vi "Efficiency Plot Main.vi"(0 "SMU 1 (Source)":refnum<k15>="4139_1", 1 "Voltage Steps":dbl[](array[numeric])=[8.5, 12.0, 24.0, 36.0, 48.0, 60.0], 5 "SMU 2 (Sink)":refnum<k15>="4139_2", 7 "Current Sweep Start":dbl format="%0.2f", 9 "Current Sweep End":dbl=-3.0 format="%0.2f", 11 "Error In":errorcluster, 12 "# Points":i32=50) -> (6 "Efficiency Plot":cluster{"current measurements":dbl[], dbl[]}[](graph)=[{"current measurements"=[0.0, 0.061224489795918366, 0.12244897959183673, 0.1836734693877551, 0.24489795918367346, 0.30612244897959184, 0.3673469387755102, 0.42857142857142855, 0.4897959183673469, 0.5510204081632653, 0.6122448979591837, 0.673469387755102, 0.7346938775510204, 0.7959183673469388, 0.8571428571428571, 0.9183673469387755, 0.9795918367346939, 1.0408163265306123, 1.1020408163265305, 1.163265306122449, 1.2244897959183674, 1.2857142857142858, 1.346938775510204, 1.4081632653061225, 1.469387755102041, 1.530612244897959, 1.5918367346938775, 1.653061224489796, 1.7142857142857142, 1.7755102040816326, 1.836734693877551, 1.8979591836734695, 1.9591836734693877, 2.020408163265306, 2.0816326530612246, 2.142857142857143, 2.204081632653061, 2.2653061224489797, 2.326530612244898, 2.3877551020408165, 2.4489795918367347, 2.510204081632653, 2.5714285714285716, 2.63265306122449, 2.693877551020408, 2.7551020408163267, 2.816326530612245, 2.877551020408163, 2.938775510204082, 3.0], [nan, inf, inf, inf, inf, inf, inf, inf, inf, inf, inf, inf, inf, inf, inf, inf, inf, inf, inf, inf, inf, inf, inf, inf, inf, inf, inf, inf, inf, inf, inf, inf, inf, inf, inf, inf, inf, inf, inf, inf, inf, inf, inf, inf, inf, inf, inf, inf, inf, inf]}, {"current measurements"=[0.0, 0.061224489795918366, 0.12244897959183673, 0.1836734693877551, 0.24489795918367346, 0.30612244897959184, 0.3673469387755102, 0.42857142857142855, 0.4897959183673469, 0.5510204081632653, 0.6122448979591837, 0.673469387755102, 0.7346938775510204, 0.7959183673469388, 0.8571428571428571, 0.9183673469387755, 0.9795918367346939, 1.0408163265306123, 1.1020408163265305, 1.163265306122449, 1.2244897959183674, 1.2857142857142858, 1.346938775510204, 1.4081632653061225, 1.469387755102041, 1.530612244897959, 1.5918367346938775, 1.653061224489796, 1.7142857142857142, 1.7755102040816326, 1.836734693877551, 1.8979591836734695, 1.9591836734693877, 2.020408163265306, 2.0816326530612246, 2.142857142857143, 2.204081632653061, 2.2653061224489797, 2.326530612244898, 2.3877551020408165, 2.4489795918367347, 2.510204081632653, 2.5714285714285716, 2.63265306122449, 2.693877551020408, 2.7551020408163267, 2.816326530612245, 2.877551020408163, 2.938775510204082, 3.0], [nan, inf, inf, inf, inf, inf, inf, inf, inf, inf, inf, inf, inf, inf, inf, inf, inf, inf, inf, inf, inf, inf, inf, inf, inf, inf, inf, inf, inf, inf, inf, inf, inf, inf, inf, inf, inf, inf, inf, inf, inf, inf, inf, inf, inf, inf, inf, inf, inf, inf]}, {"current measurements"=[0.0, 0.061224489795918366, 0.12244897959183673, 0.1836734693877551, 0.24489795918367346, 0.30612244897959184, 0.3673469387755102, 0.42857142857142855, 0.4897959183673469, 0.5510204081632653, 0.6122448979591837, 0.673469387755102, 0.7346938775510204, 0.7959183673469388, 0.8571428571428571, 0.9183673469387755, 0.9795918367346939, 1.0408163265306123, 1.1020408163265305, 1.163265306122449, 1.2244897959183674, 1.2857142857142858, 1.346938775510204, 1.4081632653061225, 1.469387755102041, 1.530612244897959, 1.5918367346938775, 1.653061224489796, 1.7142857142857142, 1.7755102040816326, 1.836734693877551, 1.8979591836734695, 1.9591836734693877, 2.020408163265306, 2.0816326530612246, 2.142857142857143, 2.204081632653061, 2.2653061224489797, 2.326530612244898, 2.3877551020408165, 2.4489795918367347, 2.510204081632653, 2.5714285714285716, 2.63265306122449, 2.693877551020408, 2.7551020408163267, 2.816326530612245, 2.877551020408163, 2.938775510204082, 3.0], [nan, inf, inf, inf, inf, inf, inf, inf, inf, inf, inf, inf, inf, inf, inf, inf, inf, inf, inf, inf, inf, inf, inf, inf, inf, inf, inf, inf, inf, inf, inf, inf, inf, inf, inf, inf, inf, inf, inf, inf, inf, inf, inf, inf, inf, inf, inf, inf, inf, inf]}, {"current measurements"=[0.0, 0.061224489795918366, 0.12244897959183673, 0.1836734693877551, 0.24489795918367346, 0.30612244897959184, 0.3673469387755102, 0.42857142857142855, 0.4897959183673469, 0.5510204081632653, 0.6122448979591837, 0.673469387755102, 0.7346938775510204, 0.7959183673469388, 0.8571428571428571, 0.9183673469387755, 0.9795918367346939, 1.0408163265306123, 1.1020408163265305, 1.163265306122449, 1.2244897959183674, 1.2857142857142858, 1.346938775510204, 1.4081632653061225, 1.469387755102041, 1.530612244897959, 1.5918367346938775, 1.653061224489796, 1.7142857142857142, 1.7755102040816326, 1.836734693877551, 1.8979591836734695, 1.9591836734693877, 2.020408163265306, 2.0816326530612246, 2.142857142857143, 2.204081632653061, 2.2653061224489797, 2.326530612244898, 2.3877551020408165, 2.4489795918367347, 2.510204081632653, 2.5714285714285716, 2.63265306122449, 2.693877551020408, 2.7551020408163267, 2.816326530612245, 2.877551020408163, 2.938775510204082, 3.0], [nan, inf, inf, inf, inf, inf, inf, inf, inf, inf, inf, inf, inf, inf, inf, inf, inf, inf, inf, inf, inf, inf, inf, inf, inf, inf, inf, inf, inf, inf, inf, inf, inf, inf, inf, inf, inf, inf, inf, inf, inf, inf, inf, inf, inf, inf, inf, inf, inf, inf]}, {"current measurements"=[0.0, 0.061224489795918366, 0.12244897959183673, 0.1836734693877551, 0.24489795918367346, 0.30612244897959184, 0.3673469387755102, 0.42857142857142855, 0.4897959183673469, 0.5510204081632653, 0.6122448979591837, 0.673469387755102, 0.7346938775510204, 0.7959183673469388, 0.8571428571428571, 0.9183673469387755, 0.9795918367346939, 1.0408163265306123, 1.1020408163265305, 1.163265306122449, 1.2244897959183674, 1.2857142857142858, 1.346938775510204, 1.4081632653061225, 1.469387755102041, 1.530612244897959, 1.5918367346938775, 1.653061224489796, 1.7142857142857142, 1.7755102040816326, 1.836734693877551, 1.8979591836734695, 1.9591836734693877, 2.020408163265306, 2.0816326530612246, 2.142857142857143, 2.204081632653061, 2.2653061224489797, 2.326530612244898, 2.3877551020408165, 2.4489795918367347, 2.510204081632653, 2.5714285714285716, 2.63265306122449, 2.693877551020408, 2.7551020408163267, 2.816326530612245, 2.877551020408163, 2.938775510204082, 3.0], [nan, inf, inf, inf, inf, inf, inf, inf, inf, inf, inf, inf, inf, inf, inf, inf, inf, inf, inf, inf, inf, inf, inf, inf, inf, inf, inf, inf, inf, inf, inf, inf, inf, inf, inf, inf, inf, inf, inf, inf, inf, inf, inf, inf, inf, inf, inf, inf, inf, inf]}, {"current measurements"=[0.0, 0.061224489795918366, 0.12244897959183673, 0.1836734693877551, 0.24489795918367346, 0.30612244897959184, 0.3673469387755102, 0.42857142857142855, 0.4897959183673469, 0.5510204081632653, 0.6122448979591837, 0.673469387755102, 0.7346938775510204, 0.7959183673469388, 0.8571428571428571, 0.9183673469387755, 0.9795918367346939, 1.0408163265306123, 1.1020408163265305, 1.163265306122449, 1.2244897959183674, 1.2857142857142858, 1.346938775510204, 1.4081632653061225, 1.469387755102041, 1.530612244897959, 1.5918367346938775, 1.653061224489796, 1.7142857142857142, 1.7755102040816326, 1.836734693877551, 1.8979591836734695, 1.9591836734693877, 2.020408163265306, 2.0816326530612246, 2.142857142857143, 2.204081632653061, 2.2653061224489797, 2.326530612244898, 2.3877551020408165, 2.4489795918367347, 2.510204081632653, 2.5714285714285716, 2.63265306122449, 2.693877551020408, 2.7551020408163267, 2.816326530612245, 2.877551020408163, 2.938775510204082, 3.0], [nan, inf, inf, inf, inf, inf, inf, inf, inf, inf, inf, inf, inf, inf, inf, inf, inf, inf, inf, inf, inf, inf, inf, inf, inf, inf, inf, inf, inf, inf, inf, inf, inf, inf, inf, inf, inf, inf, inf, inf, inf, inf, inf, inf, inf, inf, inf, inf, inf, inf]}], 15 "Error Out":errorcluster)   [LabVIEW 2014]
doc: "Demonstrates how to use triggers and events to synchronize multiple channels in Sequence source mode. Use this example to sequence multiple channels in lock-step."
uses:
  <instrlib>/niDCPower/nidcpower.llb/niDCPower Output Function.ctl
  <instrlib>/niDCPower/nidcpower.llb/niDCPower Source Mode.ctl
  <instrlib>/niDCPower/nidcpower.llb/niDCPower Sense.ctl
  <instrlib>/niDCPower/nidcpower.llb/niDCPower Sequence Attribute Type.ctl
  <instrlib>/niDCPower/nidcpower.llb/niDCPower Disable Source Trigger.vi
  <instrlib>/niDCPower/nidcpower.llb/niDCPower Configure Digital Edge Source Trigger.vi
  <instrlib>/niDCPower/nidcpower.llb/niDCPower Configure Digital Edge Measure Trigger.vi
panel:
  out "Input Voltage":cluster{"current measurements":dbl[], dbl[]}[](graph)=[{"current measurements"=[0.0037055805732003674, 0.06122110398172464, 0.12244845565372843, 0.18367430714253996, 0.24489790835656308, 0.30612338479957657, 0.3673477361051958, 0.42857227493371414, 0.48979531357904005, 0.5510198524075584, 0.6122447662818747, 0.673469305110393, 0.7346947815534065, 0.7959172576300354, 0.857143859210443, 0.9183685855618604, 0.9795921867758836, 1.0408167256044016, 1.102040139295526, 1.1632659907843375, 1.2244892169525623, 1.285714130826879, 1.3469392322240943, 1.4081635835297135, 1.4693883098811307, 1.5306113485264567, 1.5918375750610665, 1.6530617388437865, 1.7142855275807087, 1.7755106289779243, 1.8367346052377453, 1.8979597066349607, 1.9591831203260848, 2.0204080342004014, 2.0816321979831214, 2.1428574869032357, 2.204081838208855, 2.265305814468676, 2.3265305408200936, 2.387755642217309, 2.448979430954231, 2.5102045323514464, 2.571428696134167, 2.632652672393988, 2.693877586268304, 2.75510268766552, 2.8163259138337446, 2.877551390276758, 2.9387749914907815, 3.0000000928879964], [19.29819394334798, 86.6520550767066, 89.1654412635221, 91.38533524327332, 91.50919660281357, 92.04751308332489, 92.33568575131514, 92.46037426727128, 92.47606005503741, 92.42123593490287, 92.31633388123458, 92.17328677567859, 92.0042087848853, 91.81449657528333, 91.60799389168226, 91.38693943759473, 91.15523608809022, 90.91418462998905, 90.66679244318738, 90.41242663064665, 90.15379458586094, 89.89035373889821, 89.62363196341397, 89.35443181493694, 89.0829213803808, 88.80907867441277, 88.53272214141926, 88.25601431857473, 87.97816171947375, 87.69877401847535, 87.41899688296768, 87.13793625680408, 86.8562096461585, 86.57443041220006, 86.29187961010945, 86.0089768110029, 85.72632265506134, 85.4430679771896, 85.15955759219828, 84.87583568868575, 84.59217845404815, 84.30856400484413, 84.02480342907647, 83.74090983368129, 83.4569315652573, 83.17294308961198, 82.88907469498393, 82.6048754694049, 82.32014719341976, 82.03612720394379]}, {"current measurements"=[0.00021184144129742449, 0.06124941993947879, 0.12244864317662747, 0.18367468218833802, 0.24489772083366404, 0.30612282223087944, 0.36734661096780163, 0.4285726499795121, 0.4897964387164343, 0.5510209775449526, 0.6122447662818747, 0.6734694926332921, 0.7346942189847093, 0.7959183827674297, 0.8571419839814528, 0.9183672729015672, 0.9795906865926912, 1.0408157879899067, 1.102041076910021, 1.1632650531698423, 1.2244901545670577, 1.2857139433039797, 1.3469392322240943, 1.4081626459152183, 1.4693869972208375, 1.530611911095154, 1.5918370124923693, 1.6530621138895845, 1.7142855275807087, 1.775511004023722, 1.8367336676232504, 1.8979608317723549, 1.959183870417681, 2.02040634649431, 2.0816320104602224, 2.1428571118574378, 2.204080525548562, 2.265306189514474, 2.3265311033887905, 2.3877545170799146, 2.4489798060000294, 2.5102034072140524, 2.5714290711799648, 2.632653610008483, 2.693877586268304, 2.755102125096822, 2.8163259138337446, 2.877551765322556, 2.9387759291052764, 3.0000000928879964], [56.6452542558813, 80.64227031187568, 87.0782866841797, 86.4785053269065, 89.32488877347564, 88.67595189905475, 89.15300101728961, 89.59253187147004, 89.86482984693276, 90.01464408273661, 90.0842481389631, 90.0895693933995, 90.04935336193377, 89.97252157312707, 89.86619630761724, 89.73862887195637, 89.59305334468831, 89.43205240492902, 89.25985297739904, 89.07821163422473, 88.88761304096813, 88.68990824241101, 88.48605698427171, 88.2764978181229, 88.06295738097351, 87.84560283879459, 87.62562758853488, 87.40179887429976, 87.17616618084455, 86.94823753292036, 86.71826008167221, 86.4862789162294, 86.25326003643778, 86.01881763901763, 85.78341370157021, 85.54697019723872, 85.30945238666278, 85.07146384055599, 84.83237181630791, 84.59295584630685, 84.35280491363186, 84.11253310369847, 83.8713144132906, 83.63013754328348, 83.38832591662973, 83.14593896372894, 82.90348640956906, 82.66064568747939, 82.41734835561658, 82.17465456869868]}, {"current measurements"=[0.00023190639149405184, 0.06122616709999856, 0.12244845565372843, 0.18367299448224672, 0.24489790835656308, 0.30611963434159584, 0.3673464234449026, 0.4285713373192189, 0.4897964387164343, 0.5510202274533564, 0.6122443912360767, 0.6734694926332921, 0.7346936564160123, 0.7959187578132277, 0.8571427340730488, 0.9183668978557691, 0.9795916242071864, 1.0408159755128055, 1.102040889387122, 1.16326355298665, 1.2244895919983605, 1.285714130826879, 1.346939044701195, 1.4081630209610165, 1.4693877473124337, 1.5306117235722547, 1.5918360748778742, 1.6530615513208875, 1.7142855275807087, 1.775509691363429, 1.8367346052377453, 1.8979595191120617, 1.959183870417681, 2.020407096585906, 2.081631260368626, 2.1428571118574378, 2.204081463163057, 2.265305251899979, 2.3265301657742956, 2.387754892125713, 2.4489798060000294, 2.5102037822598504, 2.5714285086112674, 2.632653797531382, 2.693877961314102, 2.755102125096822, 2.8163264764024416, 2.8775504526622626, 2.93877517901368, 3.000000467933795], [24.507067975438325, 68.68728407459058, 75.82006753966498, 78.25552005826663, 80.46810288856278, 81.5286702792574, 83.9145213137586, 82.96197637388521, 83.64042372245805, 84.24184670017351, 84.68700598501955, 85.0119534280727, 85.2481904232033, 85.41356902440856, 85.52424026092518, 85.58780240316204, 85.61774812151559, 85.61373769771822, 85.58677874443494, 85.53768144152752, 85.47041365831792, 85.3885602534251, 85.29208143582215, 85.18407226185528, 85.06622105245873, 84.93930083598772, 84.80408544461643, 84.66242404506731, 84.51473417683798, 84.36085389725363, 84.2039049718862, 84.0407564161272, 83.87464336928115, 83.70526524132413, 83.53190139693746, 83.35600218690755, 83.17816187187974, 82.9976732670588, 82.81541633533251, 82.6305653803378, 82.44424776515379, 82.25691743396621, 82.06755259908867, 81.87689870447574, 81.68442031353618, 81.49075118570893, 81.29623828053742, 81.10028186493017, 80.90335145217146, 80.7055496663307]}, {"current measurements"=[0.00023828217006122054, 0.06122185407332076, 0.1224488306995265, 0.18367299448224672, 0.24489734578786596, 0.3061211345247881, 0.3673479236280948, 0.428571712365017, 0.4897960636706362, 0.5510207900220535, 0.6122449538047738, 0.673469680156191, 0.7346945940305074, 0.7959191328590258, 0.8571423590272509, 0.9183676479473653, 0.9795916242071864, 1.0408148503754115, 1.102040139295526, 1.1632652406927413, 1.2244903420899567, 1.285714318349778, 1.346938294609599, 1.4081628334381173, 1.4693868096979386, 1.5306109734806586, 1.5918364499236723, 1.6530624889353827, 1.7142851525349105, 1.775510066409227, 1.8367347927606443, 1.8979604567265569, 1.959183682894782, 2.0204087842919973, 2.0816327605518183, 2.1428571118574378, 2.2040816506859557, 2.265305814468676, 2.3265301657742956, 2.3877539545112176, 2.448979430954231, 2.5102047198743453, 2.5714273834738735, 2.63265229734819, 2.693877961314102, 2.7551017500510246, 2.816326663925341, 2.877551765322556, 2.938776491673974, 3.000000280410896], [15.625320952350052, 68.45323352659621, 68.41479018064763, 69.36918413162428, 75.8408948245319, 75.08515720349499, 78.57364834176967, 79.09049129203136, 78.79924593960071, 79.68628362365168, 80.3835328954986, 80.92405302473288, 81.34616501232134, 81.67333964560312, 81.92586994884321, 82.11470651158638, 82.25453463207786, 82.35150990030361, 82.41275896985898, 82.44583047463823, 82.45295390124451, 82.43852926466492, 82.40514186318386, 82.35672641765188, 82.2929138664694, 82.21790050512587, 82.13002218463713, 82.03354607731744, 81.92911100377732, 81.81594657215598, 81.6972655918749, 81.57150116100678, 81.44053403895059, 81.30463459966806, 81.16453795321308, 81.02039448531497, 80.87156952359493, 80.71958175528403, 80.56473166988907, 80.40678674122074, 80.2462075295369, 80.08317063844467, 79.91912233101111, 79.75064757843249, 79.58076401285685, 79.41032236358052, 79.23731818637971, 79.06327995782223, 78.88659495956507, 78.70957354063141]}, {"current measurements"=[0.0002388447387583213, 0.061227104714493726, 0.12244620537894002, 0.1836713067761554, 0.24490147129164477, 0.30612732278045623, 0.36734979885708513, 0.4285707747505218, 0.4897960636706362, 0.5510209775449526, 0.6122449538047738, 0.673468742541696, 0.7346945940305074, 0.7959187578132277, 0.8571429215959478, 0.91836671033287, 0.9795916242071864, 1.0408163505586037, 1.10204126443292, 1.1632656157385395, 1.2244910921815528, 1.285714130826879, 1.346938857178296, 1.4081624583923191, 1.4693881223582317, 1.530613598801245, 1.591835887354975, 1.6530611762750895, 1.7142855275807087, 1.775510816500823, 1.8367342301919474, 1.8979587690204656, 1.959183682894782, 2.0204085967690983, 2.0816323855060204, 2.1428574869032357, 2.20408090059436, 2.265306001991575, 2.3265297907284976, 2.3877547046028136, 2.448978868385534, 2.510203032168254, 2.571428883657066, 2.632652672393988, 2.6938772112225062, 2.7551023126197216, 2.816327414016937, 2.8775510152309596, 2.9387755540594784, 3.000000842979593], [10.685809147475581, 60.58664973802159, 69.32426572969297, 70.02017096472375, 70.60628775716478, 69.48609512689428, 73.16747403099501, 75.51894590720678, 74.45380140438738, 75.42803512625773, 76.3187834034888, 77.02711378666972, 77.591621229274, 78.04913495784959, 78.41201146737268, 78.7051508644127, 78.93314890895036, 79.11244376640121, 79.24599906988342, 79.3472307513215, 79.41532553446862, 79.45725266090052, 79.47501728817076, 79.47396673288904, 79.45412055016777, 79.41874717833805, 79.36947408129463, 79.30858436763418, 79.23748643871782, 79.15581950747247, 79.06485359860626, 78.96714312929933, 78.86342088702459, 78.75295744414646, 78.63548168504948, 78.51333325794127, 78.38617989431057, 78.25366220787029, 78.11974624015173, 77.98035710245406, 77.83837311795462, 77.69253126803493, 77.54419990931002, 77.39221211507345, 77.2389193042367, 77.08179535393343, 76.92307638925759, 76.76351534955948, 76.60023763509811, 76.43545824058003]}, {"current measurements"=[0.00023996987615252285, 0.061227104714493726, 0.12243795437138254, 0.18367468218833802, 0.24489997110845244, 0.30611813415840355, 0.3673460483991045, 0.42857096227342084, 0.4897926882584537, 0.5510215401136497, 0.6122455163734709, 0.6734700552019891, 0.7346947815534065, 0.7959180077216316, 0.8571429215959478, 0.9183674604244662, 0.9795919992529845, 1.0408165380815027, 1.102041076910021, 1.1632650531698423, 1.2244890294296633, 1.285713755781081, 1.3469375445180027, 1.4081637710526127, 1.4693866221750393, 1.53061266118675, 1.5918370124923693, 1.6530600511376952, 1.7142864651952041, 1.775510066409227, 1.8367347927606443, 1.8979595191120617, 1.959183870417681, 2.020407471631704, 2.0816335106434147, 2.1428572993803368, 2.204082025731754, 2.2653063770373736, 2.3265305408200936, 2.3877543295570156, 2.448979243431332, 2.5102049073972448, 2.5714285086112674, 2.632653234962685, 2.693877961314102, 2.7551008124365293, 2.816326663925341, 2.877551952845455, 2.938774428922084, 2.999999717842199], [8.037505223161133, 59.04402746018973, 65.93397111865757, 69.10832461216576, 69.88132934827026, 70.40864376659275, 71.07244623688928, 71.61813446388392, 70.88559085363639, 71.27919739280526, 72.31262277678016, 73.15099339025103, 73.83517876691829, 74.38997807165609, 74.8469795829111, 75.21574450005743, 75.51758140567794, 75.75633244380813, 75.94946682291643, 76.10238026373673, 76.21748823541188, 76.30401119763542, 76.36128741226422, 76.39717578408371, 76.4112319455966, 76.40815492818933, 76.38863918175531, 76.35552208706163, 76.31078311855917, 76.25546527873904, 76.18851950750565, 76.11259322339771, 76.02782989417233, 75.93726786864158, 75.84032284746705, 75.7354997513752, 75.62599197868968, 75.51069814477592, 75.39257747375275, 75.2695297016027, 75.14021925250529, 75.00917395178712, 74.87370939203441, 74.7357885393685, 74.59436663020796, 74.45166513872823, 74.30470438952655, 74.15585812945028, 74.00505290512945, 73.85269262177381]}]
  # "Sink"
  # "SOURCING OPERATION (SMU 1)\n1. Source Voltage Level and Fire Source Trigger Event \n2. Wait \"Delay\" Seconds\n3. Fire Source Complete Event\n3. Measure Current Immediately\n\nIV1, IV2, IV3...IV300 at V IN"
  # "SINKING OPERATION (SMU 2)\n1. Source Current Level (SMU1 Trigger)\n2. Wait \"Delay\" Seconds\n3. Measure Voltage (Using SMU1 Source Complete Event Trigger)\n\n\nIV1, IV2, IV3...IV300 at V OUT"
  # "Source"
  # "Iout = 0 to 3 A"
  # "Vin = 8 to 60 V"
  # "Vout = 5 V"
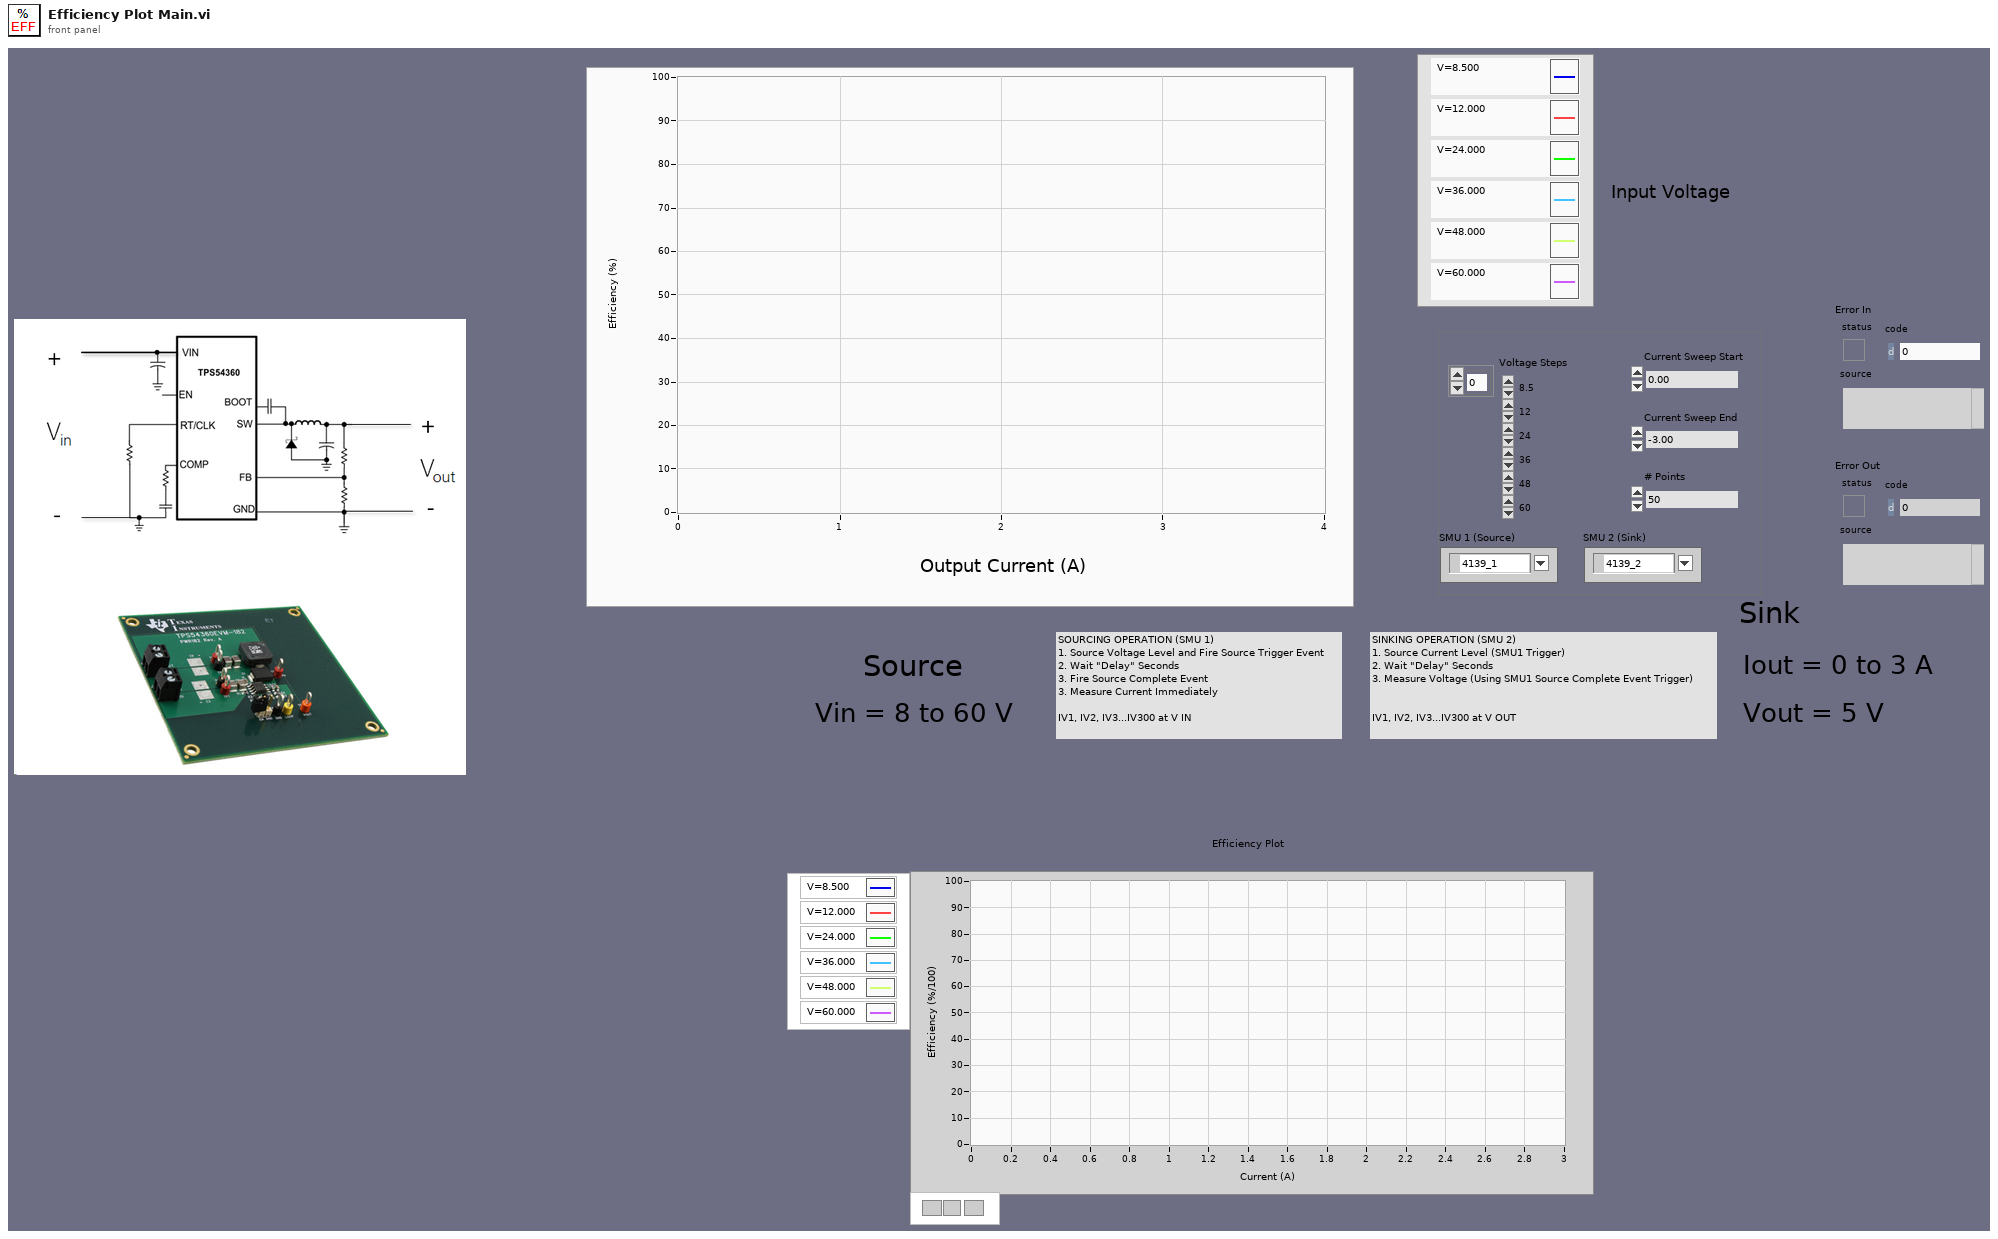
[diagram p1: front panel]
types:
  T1 = typedef "niDCPower Sequence Attribute Type.ctl" = i32
  T2 = typedef "niDCPower Sense.ctl" = i32
  T3 = typedef "niDCPower Source Mode.ctl" = i32
  T4 = typedef "niDCPower Output Function.ctl" = i32
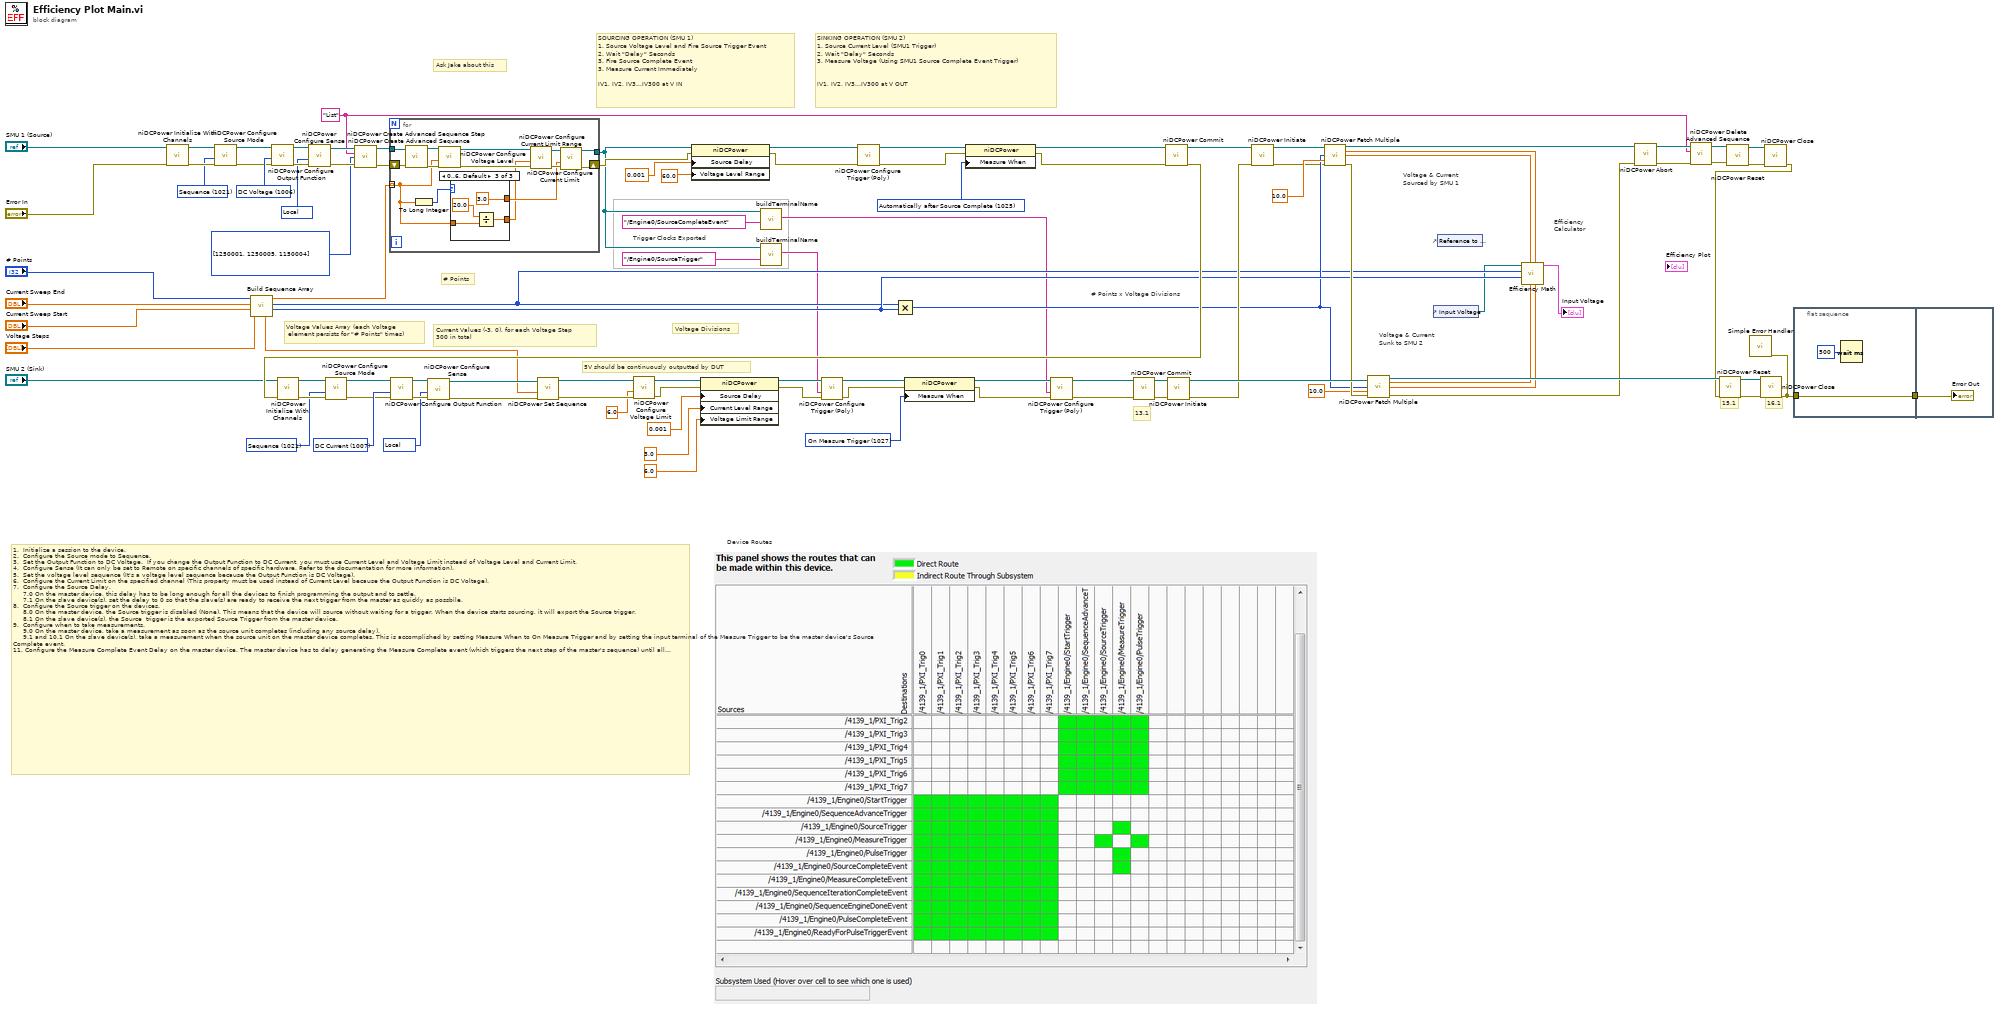
[diagram p0: block diagram]
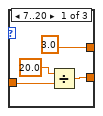
[diagram p2: hidden frame]
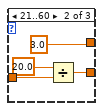
[diagram p3: hidden frame]
diagram:
  w5 = "List" ("list name")
  w20 = T1[] [1250001, 1250005, 1150004] items=["Voltage Pole-Zero Ratio"=1150069, "Voltage Compensation Frequency"=1150068, "Voltage Gain Bandwidth"=1150067, "Transient Response"=1150062, "Output Resistance"=1150061, "Output Connected"=1150060, "Output Enabled"=1250006, "Output Function"=1150008, "Source Delay"=1150051, "Aperture Time Units"=1150059, "Aperture Time"=1150058, "Voltage Limit Range"=1150012, "Voltage Limit"=1150010, "Current Level Range"=1150011, "Current Level"=1150009, "Current Limit Range"=1150004, "Current Limit"=1250005, "Voltage Level Range"=1150005, "Voltage Level"=1250001]
  w53 = T2 1008 items=["Local"=1008, "Remote"=1009] ("sense")
  w54 = T2 1008 items=["Local"=1008, "Remote"=1009] ("sense")
  w66 = 1027 items=["Automatically after Source Complete"=1025, "On Demand"=1026, "On Measure Trigger"=1027] ("Measurement:Advanced:Measure When")
  w67 = T3 1021 items=["Single Point"=1020, "Sequence"=1021] ("source mode")
  w78 = T4 1007 items=["DC Voltage"=1006, "DC Current"=1007] ("output function")
  w87 = 1025 items=["Automatically after Source Complete"=1025, "On Demand"=1026, "On Measure Trigger"=1027] ("Measurement:Advanced:Measure When")
  w88 = T3 1021 items=["Single Point"=1020, "Sequence"=1021] ("source mode")
  w95 = T4 1006 items=["DC Voltage"=1006, "DC Current"=1007] ("output function")
  # "Trigger Clocks Exported"
  # "Device Routes"
  # "Efficiency\nCalculator"
  # "Voltage & Current \nSourced by SMU 1"
  # "Voltage & Current \nSunk to SMU 2"
  # "# Points x Voltage Divisions"
  # "Ask Jake about this"
  # "SINKING OPERATION (SMU 2)\n1. Source Current Level (SMU1 Trigger)\n2. Wait \"Delay\" Seconds\n3. Measure Voltage (Using SMU1 Source Complete Event Trigger)\n\n\nIV1, IV2, IV3...IV300 at V OUT"
  # "SOURCING OPERATION (SMU 1)\n1. Source Voltage Level and Fire Source Trigger Event \n2. Wait \"Delay\" Seconds\n3. Fire Source Complete Event\n3. Measure Current Immediately\n\nIV1, IV2, IV3...IV300 at V IN"
  # "Voltage Divisions"
  # "# Points"
  # "5V should be continuously outputted by DUT"
  # "Voltage Values Array (each Voltage\n element persists for \"# Points\" times)"
  # "Current Values (-3, 0), for each Voltage Step\n300 in total"
  # "16.1"
  # "15.1"
  # "13.1"
  # "1.  Initialize a session to the device.\n2.  Configure the Source mode to Sequence.\n3.  Set the Output Function to DC Voltage.  If you change the Output Function to DC Current, you must use Current Level and Voltage Limit instead of Voltage Level and Current Limit.\n4.  Configure Sense (It can only be set to Remote on specific channels of specific hardware. Refer to the documentation for more information).\n5.  Set the voltage level sequence (It's a voltage level sequence because the Output Function is DC Voltage).\n6.  Configure the Current Limit on the specified channel (This property must be used instead of Current Level because the Output Function is DC Voltage).\n7.  Configure the Source Delay.\n     7.0 On the master device, this delay has to be long enough for all the devices to finish programming the output and to settle.\n     7.1 On the slave device(s), set the delay to 0 so that the slave(s) are ready to receive the next trigger from the master as quickly as possbile.\n8.  Configure the Source trigger on the devices.\n     8.0 On the master device, the Source trigger is disabled (None). This means that the device will source without waiting for a trigger. When the device starts sourcing, it will export the Source trigger.\n     8.1 On the slave device(s), the Source  trigger is the exported Source Trigger from the master device.\n9.  Configure when to take measurements.\n     9.0 On the master device, take a measurement as soon as the source unit completes (including any source delay).\n     9.1 and 10.1 On the slave device(s), take a measurement when the source unit on the master device completes. This is accomplished by setting Measure When to On Measure Trigger and by setting the input terminal of the Measure Trigger to be the master device's Source Complete event.\n11. Configure the Measure Complete Event Delay on the master device. The master device has to delay generating the Measure Complete event (which triggers the next step of the master's sequence) until all slave device(s) have completed taking measurements. The amount of time a slave takes to measure can vary based on its configuration and model.\n12. Commit the settings to the device so that the driver establishes all the routing required for the configured triggers and events."
  n1 = call <instrlib>:"niDCPower Initialize With Channels.vi"("error in (no error)"="Error In", "resource name"="SMU 1 (Source)") -> ("error out"=w92:errorcluster, "instrument handle out"=w89:refnum<k15>)  [unwired: 2 in, 6 out]
  n2 = call <instrlib>:"niDCPower Configure Source Mode.vi"("error in (no error)"=w92, "source mode"=w88, "instrument handle"=w89) -> ("error out"=w91:errorcluster, "instrument handle out"=w90:refnum<k15>)  [unwired: 7 out]
  n3 = call "Build Sequence Array.vi"("Voltage Steps"="Voltage Steps", "Current Sweep Start"="Current Sweep Start", "Current Sweep End"="Current Sweep End", "# Points"="# Points") -> ("# Voltage Divisions"=w35:i32, "# of Points"=w30:i32, "To SMU 1 (Source)"=w29:dbl[], "To SMU 2 (Sink)"=w28:dbl[])  [unwired: 4 in]
  n4 = call <instrlib>:"niDCPower Configure Output Function.vi"("error in (no error)"=w91, "output function"=w95, "instrument handle"=w90) -> ("error out"=w97:errorcluster, "instrument handle out"=w96:refnum<k15>)  [unwired: 1 in, 6 out]
  n5 = call <instrlib>:"niDCPower Configure Sense.vi"("error in (no error)"=w97, "sense"=w53, "instrument handle"=w96) -> ("error out"=w23:errorcluster, "instrument handle out"=w24:refnum<k15>)  [unwired: 1 in, 6 out]
  n6 = call <instrlib>:"niDCPower Create Advanced Sequence.vi"("instrument handle"=w24, "sequence name"=w5, "advanced sequence properties"=w20, "error in (no error)"=w23) -> ("instrument handle out"=w21:refnum<k15>, "error out"=w22:errorcluster)  [unwired: 10 in]
  n7 = for {
    tunnel: w21 -> [w107]
    tunnel: [w111] -> w17
    shift-right: [w110] -> w36
    shift-left: w22 -> [w104]
    tunnel: w29 -> [w103] mode=indexing
    n8 = call <instrlib>:"niDCPower Create Advanced Sequence Step.vi"("error in (no error)"=w104, "instrument handle"=w107) -> ("error out"=w105:errorcluster, "instrument handle out"=w106:refnum<k15>)  [unwired: 8 in]
    n9 = To Long Integer(number=w103) -> (32bit integer=w102:i32)
    n10 = call <instrlib>:"niDCPower Configure Voltage Level.vi"("error in (no error)"=w105, "voltage level"=w103, "instrument handle"=w106) -> ("error out"=w115:errorcluster, "instrument handle out"=w114:refnum<k15>)  [unwired: 7 in]
    n11 = case shown="0..6, Default" w102 {
      tunnel: [3.0 3.0 3.0] -> w109
      tunnel: w103 -> [w117 w120 w126]
      tunnel: [w116 w122 w124] -> w108
      frame 7..20 {
        n12 = Divide(x=20.0, y=w117) -> (x/y=w116:dbl)
      }
      frame 21..60 {
        n13 = Divide(x=20.0, y=w120) -> (x/y=w122:dbl)
      }
      frame 0..6, Default {
        n14 = Divide(x=20.0, y=w126) -> (x/y=w124:dbl)
      }
    }
    n15 = call <instrlib>:"niDCPower Configure Current Limit.vi"("error in (no error)"=w115, "current limit"=w108, "instrument handle"=w114) -> ("error out"=w112:errorcluster, "instrument handle out"=w113:refnum<k15>)  [unwired: 2 in, 5 out]
    n16 = call <instrlib>:"niDCPower Configure Current Limit Range.vi"("error in (no error)"=w112, "current limit range"=w109, "instrument handle"=w113) -> ("error out"=w110:errorcluster, "instrument handle out"=w111:refnum<k15>)  [unwired: 7 in]
  }
  n17 = property class="niDCPower"(reference=w17, error in=w36, "Source Delay"=0.001 ("Source:Advanced:Source Delay"), "Voltage Level Range"=60.0 ("Source:Advanced:Source Delay")) -> (reference out=w33:refnum<k15>, error out=w32:errorcluster)
  n18 = call "buildTerminalName.vi"("Local Terminal Name"="/Engine0/SourceCompleteEvent", "session handle"=w17) -> ("Fully Qualified Terminal Name"=w18:string)  [unwired: 7 in, 2 out]
  n19 = call "buildTerminalName.vi"("Local Terminal Name"="/Engine0/SourceTrigger", "session handle"=w17) -> ("Fully Qualified Terminal Name"=w4:string)  [unwired: 7 in, 2 out]
  n20 = call-poly <instrlib>:"niDCPower Configure Trigger (Poly).vi"("error in (no error)"=w32, "instrument handle"=w33) -> ("error out"=w93:errorcluster, "instrument handle out"=w94:refnum<k15>)  [unwired: 1 in, 7 out]
  n21 = Multiply(x=w30, y=w35) -> (x*y=w34:i32)
  n22 = property class="niDCPower"(reference=w94, error in=w93, "Measure When"=w87) -> (reference out=w82:refnum<k15>, error out=w81:errorcluster)
  n23 = call <instrlib>:"niDCPower Commit.vi"("error in (no error)"=w81, "instrument handle"=w82) -> ("error out"=w84:errorcluster, "instrument handle out"=w85:refnum<k15>)  [unwired: 8 out]
  n24 = call <instrlib>:"niDCPower Initialize With Channels.vi"("error in (no error)"=w84, "resource name"="SMU 2 (Sink)") -> ("error out"=w71:errorcluster, "instrument handle out"=w68:refnum<k15>)  [unwired: 2 in, 6 out]
  n25 = call <instrlib>:"niDCPower Configure Source Mode.vi"("error in (no error)"=w71, "source mode"=w67, "instrument handle"=w68) -> ("error out"=w70:errorcluster, "instrument handle out"=w69:refnum<k15>)  [unwired: 7 out]
  n26 = call <instrlib>:"niDCPower Configure Output Function.vi"("error in (no error)"=w70, "output function"=w78, "instrument handle"=w69) -> ("error out"=w80:errorcluster, "instrument handle out"=w79:refnum<k15>)  [unwired: 1 in, 6 out]
  n27 = call <instrlib>:"niDCPower Configure Sense.vi"("error in (no error)"=w80, "sense"=w54, "instrument handle"=w79) -> ("error out"=w76:errorcluster, "instrument handle out"=w77:refnum<k15>)  [unwired: 1 in, 6 out]
  n28 = call <instrlib>:"niDCPower Set Sequence.vi"("error in (no error)"=w76, "values"=w28, "instrument handle"=w77) -> ("error out"=w62:errorcluster, "instrument handle out"=w63:refnum<k15>)  [unwired: 2 in, 5 out]
  n29 = call <instrlib>:"niDCPower Configure Voltage Limit.vi"("error in (no error)"=w62, "voltage limit"=6.0, "instrument handle"=w63) -> ("error out"=w61:errorcluster, "instrument handle out"=w60:refnum<k15>)  [unwired: 7 in]
  n30 = property class="niDCPower"(reference=w60, error in=w61, "Source Delay"=0.001 ("Source:Advanced:Source Delay"), "Current Level Range"=3.0 ("Source:Advanced:Source Delay"), "Voltage Limit Range"=6.0 ("Source:Advanced:Source Delay")) -> (reference out=w64:refnum<k15>, error out=w65:errorcluster)
  n31 = call-poly <instrlib>:"niDCPower Configure Trigger (Poly).vi"("error in (no error)"=w65, "input terminal"=w4, "instrument handle"=w64) -> ("error out"=w74:errorcluster, "instrument handle out"=w75:refnum<k15>)  [unwired: 1 in, 6 out]
  n32 = property class="niDCPower"(reference=w75, error in=w74, "Measure When"=w66) -> (reference out=w72:refnum<k15>, error out=w73:errorcluster)
  n33 = call-poly <instrlib>:"niDCPower Configure Trigger (Poly).vi"("error in (no error)"=w73, "input terminal"=w18, "instrument handle"=w72) -> ("error out"=w51:errorcluster, "instrument handle out"=w52:refnum<k15>)  [unwired: 1 in, 6 out]
  n34 = call <instrlib>:"niDCPower Commit.vi"("error in (no error)"=w51, "instrument handle"=w52) -> ("error out"=w99:errorcluster, "instrument handle out"=w100:refnum<k15>)  [unwired: 8 out]
  n35 = call <instrlib>:"niDCPower Initiate.vi"("error in (no error)"=w99, "instrument handle"=w100) -> ("error out"=w86:errorcluster, "instrument handle out"=w101:refnum<k15>)  [unwired: 8 out]
  n36 = call <instrlib>:"niDCPower Initiate.vi"("error in (no error)"=w86, "instrument handle"=w85) -> ("error out"=w27:errorcluster, "instrument handle out"=w26:refnum<k15>)  [unwired: 8 out]
  n37 = call <instrlib>:"niDCPower Fetch Multiple.vi"("instrument handle"=w26, "count (1)"=w34, "timeout (sec)"=10.0, "error in (no error)"=w27) -> ("instrument handle out"=w11:refnum<k15>, "voltage measurements"=w43:dbl[], "current measurements"=w44:dbl[], "error out"=w83:errorcluster)  [unwired: 1 in, 7 out]
  n38 = call <instrlib>:"niDCPower Fetch Multiple.vi"("instrument handle"=w101, "count (1)"=w34, "timeout (sec)"=10.0, "error in (no error)"=w83) -> ("instrument handle out"=w98:refnum<k15>, "voltage measurements"=w45:dbl[], "current measurements"=w42:dbl[], "error out"=w12:errorcluster)  [unwired: 1 in, 7 out]
  n39 = control-ref of="Input Voltage"() -> (w2:refnum<vi>)
  n40 = control-ref of="Reference to XY Graph"() -> ()  [unwired: 1 out]
  n41 = call "Efficiency Math.vi"("SMU 2 Current Measurements"=w42, "SMU 1 Voltage Measurements"=w43, "SMU 2 Voltage Measurements"=w45, "SMU 1 Current Measurements"=w44, "# Voltage Divisions"=w35, "# Points"=w30, "XYGraph in"=w2) -> ("Array"=→"Input Voltage":cluster{"Array":dbl[], "Array":dbl[]}[])  [unwired: 4 in]
  n42 = call <instrlib>:"niDCPower Abort.vi"("error in (no error)"=w12, "instrument handle"=w11) -> ("error out"=w7:errorcluster, "instrument handle out"=w10:refnum<k15>)  [unwired: 8 in]
  n43 = call <instrlib>:"niDCPower Delete Advanced Sequence.vi"("error in (no error)"=w7, "sequence name"=w5, "instrument handle"=w10) -> ("error out"=w8:errorcluster, "instrument handle out"=w9:refnum<k15>)  [unwired: 7 in]
  n44 = call <instrlib>:"niDCPower Reset.vi"("error in (no error)"=w8, "instrument handle"=w9) -> ("error out"=w15:errorcluster, "instrument handle out"=w14:refnum<k15>)  [unwired: 1 in, 7 out]
  n45 = call <instrlib>:"niDCPower Close.vi"("error in (no error)"=w15, "instrument handle"=w14) -> ("error out"=w6:errorcluster)  [unwired: 9 out]
  n46 = call <instrlib>:"niDCPower Reset.vi"("error in (no error)"=w6, "instrument handle"=w98) -> ("error out"=w59:errorcluster, "instrument handle out"=w58:refnum<k15>)  [unwired: 1 in, 7 out]
  n47 = call <instrlib>:"niDCPower Close.vi"("error in (no error)"=w59, "instrument handle"=w58) -> ("error out"=w13:errorcluster)  [unwired: 9 out]
  n48 = call <vilib>:"Simple Error Handler.vi"("error in (no error)"=w13) -> ()  [unwired: 4 in, 5 out]
  n49 = flat-sequence {
    tunnel: w13 -> [w129]
    tunnel: [w129] -> w3
    tunnel: w3 -> [w130]
    frame #0 {
      n50 = Wait (ms)(milliseconds to wait=u32 500) -> ()  [unwired: 1 out]
    }
    frame #1 {
      "Error Out" <- w130
    }
  }
